vi "gds_top_simulator.vi"() -> ()   [LabVIEW 2012]
uses:
  EE 497/LABS/SDR/control_type_defs.llb/tx_hw params.ctl
  EE 497/LABS/SDR/control_type_defs.llb/rx_hw params.ctl
panel:
  out "Q":waveform(dbl)(graph)
  out "I":waveform(dbl)(graph)
  out "average \nbit-error rate":dbl
  in  "stop":bool
  out "error out":errorcluster
  in  "error in":errorcluster
  out "bit-error rate":dbl
  in  "RX Parameters":T1={"Sampling Rate"=4000000.0, "RX Oversample Factor"=4}
  in  "Shared Parameters":T2={"Packet Length"=500, "Preamble Length"=20, "modulation type"=enum."OOK", "FSK deviation (Hz)"=625.0, "Filter Parameters"={"modulation type"=enum."ASK", "pulse shaping filter (none)"=enum."none", "filter length (symbols)"=8, "filter parameter"=0.5}}
  in  "TX Parameters":T3={"Sampling Rate"=4000000.0, "Oversample Factor"=4} {"Sampling Rate" format="%^.2e"}
  in  "Channel Model Parameters":T4={"Channel Type"=enum."Gaussian", "Noise Power (dB)"=-inf, "Channel Response"=[], "Frequency Offset (Hz)"=0.0, "Delay (s)"=0.0}
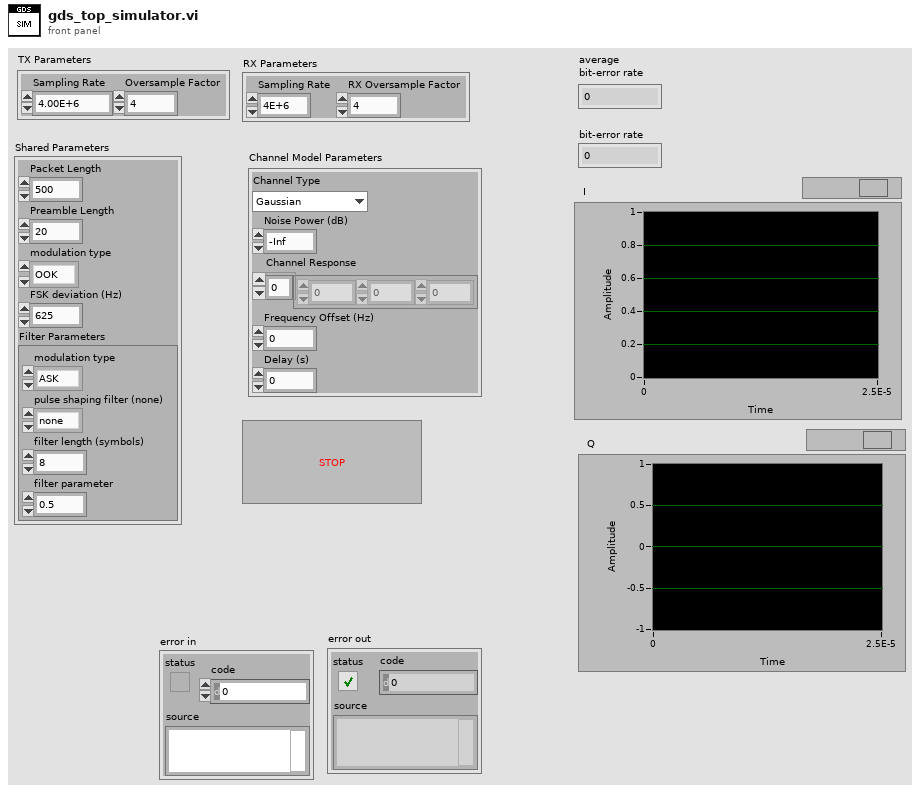
[diagram p1: front panel]
types:
  T1 = cluster{"Sampling Rate":dbl, "RX Oversample Factor":i32}
  T2 = cluster{"Packet Length":i32, "Preamble Length":i32, "modulation type":enum16{"OOK", "FSK", "PSK", "QAM", "MSK", "PAM", "ASK", "CPM"}, "FSK deviation (Hz)":dbl, "Filter Parameters":cluster{"modulation type":enum16{"FSK", "PSK", "QAM", "MSK", "PAM", "ASK", "CPM"}, "pulse shaping filter (none)":enum16{"none", "Raised Cosine", "Root Raised Cos", "Gaussian"}, "filter length (symbols)":i32, "filter parameter":dbl}}
  T3 = cluster{"Sampling Rate":dbl, "Oversample Factor":i32}
  T4 = cluster{"Channel Type":enum16{"Gaussian", "ISI"}, "Noise Power (dB)":dbl, "Channel Response":cdb[], "Frequency Offset (Hz)":dbl, "Delay (s)":dbl}
  T5 = typedef "rx_hw params.ctl" = cluster{"Device IP Address":refnum<k15>, "Active Antenna":string, "Carrier Frequency (Hz)":dbl, "Gain (dB)":dbl, "Trigger Level":dbl, "Bandwidth (Hz)":dbl, "Reference Position (%)":dbl, "Capture Time (s)":dbl, "Simulate":bool}
  T6 = typedef "tx_hw params.ctl" = cluster{"Device IP Address":refnum<k15>, "Active Antenna":string, "Carrier Frequency (Hz)":dbl, "Gain (dB)":dbl, "Generation Mode":enum16{"single shot", "simulate", "continuous"}}
  T7 = cluster{"TX Parameters":cluster{"Sampling Rate":dbl, "Oversample Factor":i32}, "Shared Parameters":cluster{"Packet Length":i32, "Preamble Length":i32, "modulation type":enum16{"OOK", "FSK", "PSK", "QAM", "MSK", "PAM", "ASK", "CPM"}, "FSK deviation (Hz)":dbl, "Filter Parameters":cluster{"modulation type":enum16{"FSK", "PSK", "QAM", "MSK", "PAM", "ASK", "CPM"}, "pulse shaping filter (none)":enum16{"none", "Raised Cosine", "Root Raised Cos", "Gaussian"}, "filter length (symbols)":i32, "filter parameter":dbl}}}
  T8 = typedef "niAMT.lvlib/Complex Data Waveform.ctl" = cluster{"t0":dbl, "dt":dbl, "Y":cdb[]}
  T9 = cluster{"RX Parameters":cluster{"Sampling Rate":dbl, "RX Oversample Factor":i32}, "Shared Parameters":cluster{"Packet Length":i32, "Preamble Length":i32, "modulation type":enum16{"OOK", "FSK", "PSK", "QAM", "MSK", "PAM", "ASK", "CPM"}, "FSK deviation (Hz)":dbl, "Filter Parameters":cluster{"modulation type":enum16{"FSK", "PSK", "QAM", "MSK", "PAM", "ASK", "CPM"}, "pulse shaping filter (none)":enum16{"none", "Raised Cosine", "Root Raised Cos", "Gaussian"}, "filter length (symbols)":i32, "filter parameter":dbl}}}
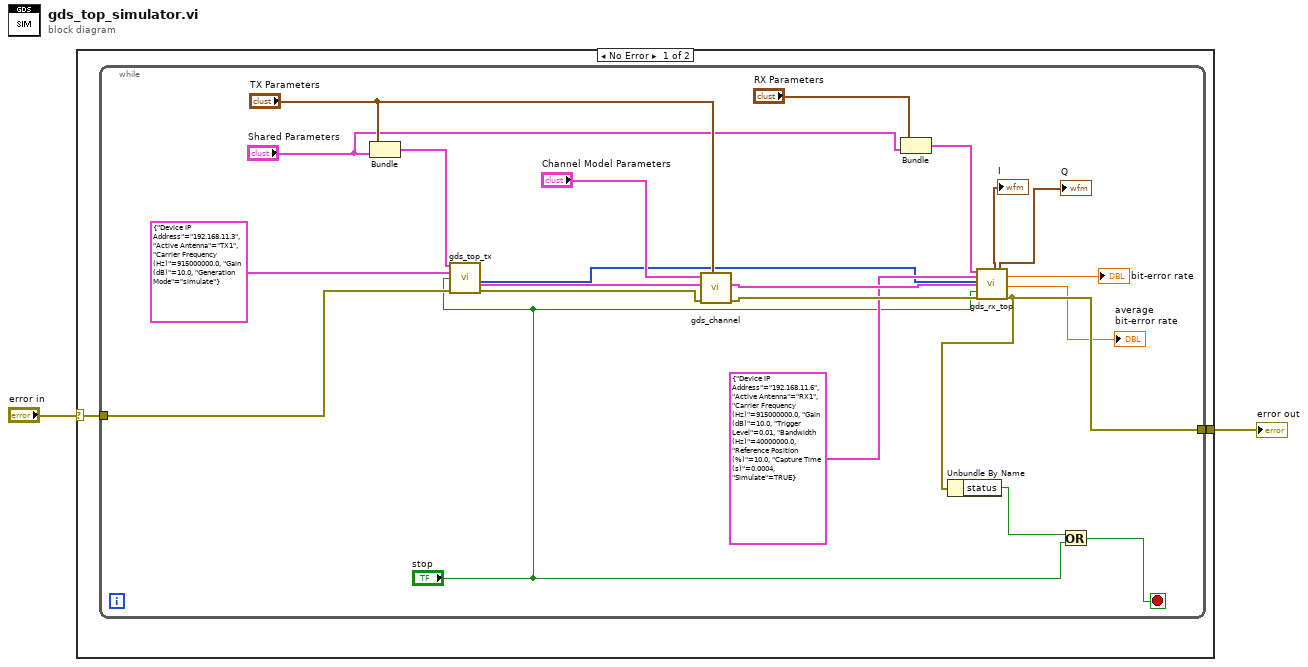
[diagram p0: block diagram]
diagram:
  n1 = case shown="No Error" "error in" {
    selector: "error in" -> [w3 w27]
    tunnel: [w4 w27] -> w2
    frame No Error {
      n2 = while {
        tunnel: [w11] -> w4
        tunnel: w3 -> [w12]
        stop <- w8 stop-if-true
        n3 = Bundle("TX Parameters"="TX Parameters", "Shared Parameters"="Shared Parameters") -> (w20:T7)  [unwired: 1 in]
        n4 = call "gds_top_tx.vi"("Modulation Parameters"=w20, "HW parameters In"=T6 {"Device IP Address"="192.168.11.3", "Active Antenna"="TX1", "Carrier Frequency (Hz)"=915000000.0, "Gain (dB)"=10.0, "Generation Mode"=enum."simulate"}, "STOP"="stop", "error in"=w12) -> ("key bit sequence"=w13:i8[], "output IQ waveform"=w26:cluster{"t0":dbl, "dt":dbl, "Y":cdb[]}, "error out"=w24:errorcluster)  [unwired: 1 in, 8 out]
        n5 = call "gds_channel.vi"("TX Parameters"="TX Parameters", "error in (no error)"=w24, "input complex waveform"=w26, "Channel Model Parameters"="Channel Model Parameters") -> ("error out"=w23:errorcluster, "output complex waveform"=w25:T8)  [unwired: 6 in]
        n6 = Bundle("RX Parameters"="RX Parameters", "Shared Parameters"="Shared Parameters") -> (w17:T9)  [unwired: 1 in]
        n7 = call "gds_rx_top.vi"("Modulation Parameters"=w17, "HW parameters"=T5 {"Device IP Address"="192.168.11.6", "Active Antenna"="RX1", "Carrier Frequency (Hz)"=915000000.0, "Gain (dB)"=10.0, "Trigger Level"=0.01, "Bandwidth (Hz)"=40000000.0, "Reference Position (%)"=10.0, "Capture Time (s)"=0.0004, "Simulate"=TRUE}, "Received Bit Sequence"=w13, "Received IQ\nwaveform"=w25, "stop"="stop", "error in"=w23) -> ("I"=→"I":waveform(dbl), "Q"=→"Q":waveform(dbl), "bit-error rate"=→"bit-error rate":dbl, "average \nbit-error rate"=→"average \nbit-error rate":dbl, "error out"=w11:errorcluster)  [unwired: 4 in, 5 out]
        n8 = Unbundle By Name(w11) -> ("status"=w10:bool)
        n9 = Or(x=w10, y="stop") -> (x .or. y?=w8:bool)
      }
    }
    frame Error {
    }
  }
  "error out" <- w2
